vi "Get Service Descriptor.vi"(8 "error in":errorcluster) -> (0 "error out":errorcluster, 3 "service descriptor":T1)   [LabVIEW 2022 SP3, in "Single Tone - Digital Mic.lvlib"]
uses:
  Single Tone - Digital Mic.lvlib
  <vilib>/Plug-In SDKs/Measurements/Helpers/TypeDefs/Service Descriptor.ctl
  <vilib>/Plug-In SDKs/Measurements/Helpers/TypeDefs/Measurement Details.ctl
  <vilib>/Plug-In SDKs/Measurements/Helpers/TypeDefs/Measurement Annotation.ctl
  <vilib>/Plug-In SDKs/Measurements/NI Measurement Plug-In SDK.lvlib
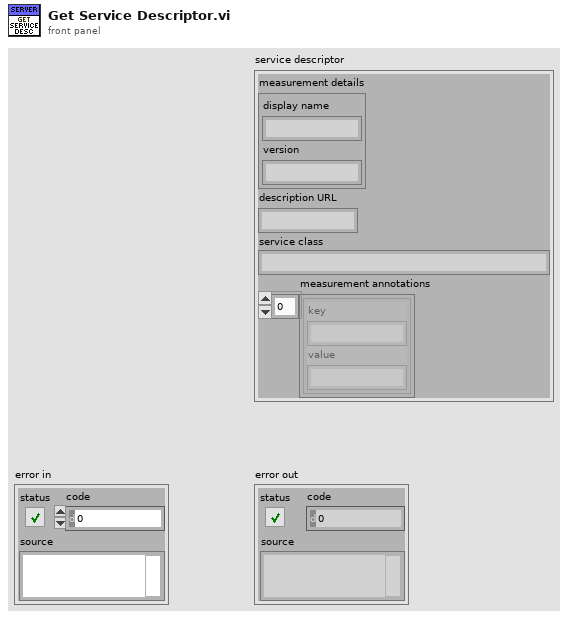
[diagram p1: front panel]
types:
  T1 = typedef "NI Measurement Plug-In SDK.lvlib/Service Descriptor.ctl" = cluster{"measurement details":T2, "description URL":string, "service class":string, "measurement annotations":T3[]}
  T2 = typedef "NI Measurement Plug-In SDK.lvlib/Measurement Details.ctl" = cluster{"display name":string, "version":string}
  T3 = typedef "NI Measurement Plug-In SDK.lvlib/Measurement Annotation.ctl" = cluster{"key":string, "value":string}
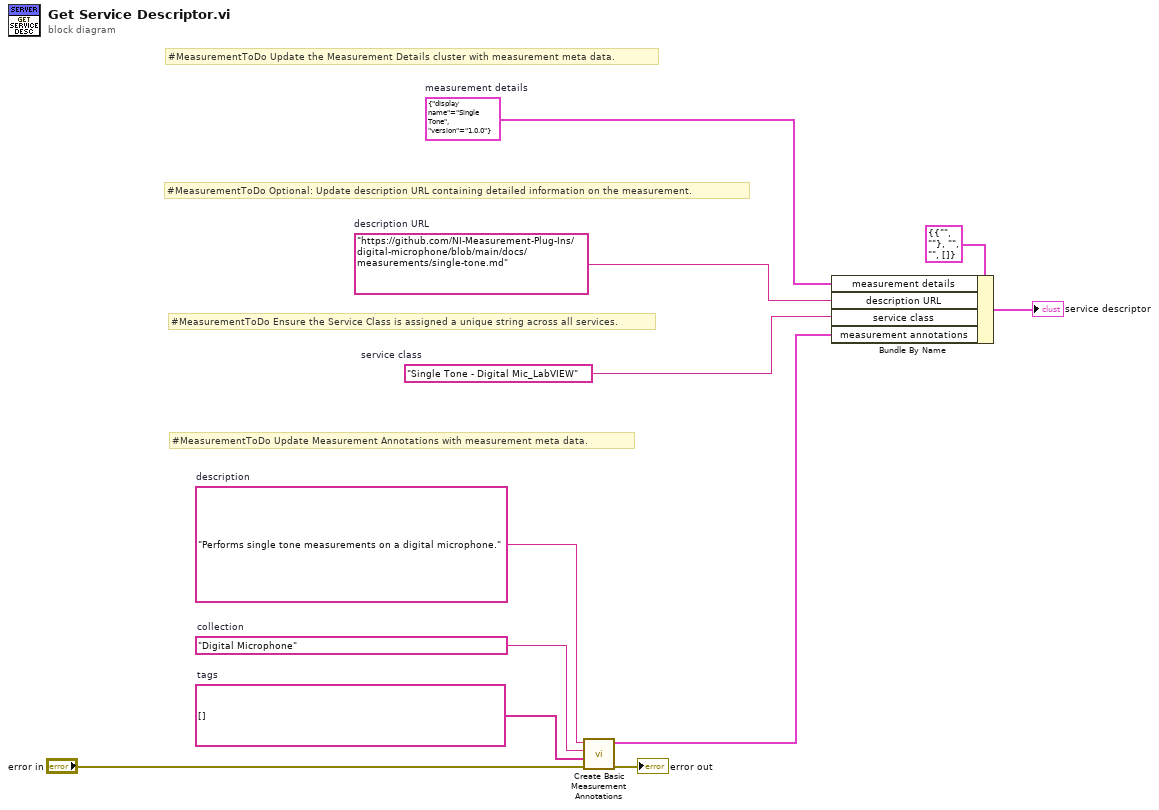
[diagram p0: block diagram]
diagram:
  w5 = "https://github.com/NI-Measurement-Plug-Ins/digital-microphone/blob/main/docs/measurements/single-tone.md"  # description URL
  w7 = string[] []  # tags
  w8 = "Digital Microphone"  # collection
  w9 = "Performs single tone measurements on a digital microphone."  # description
  w6 = T2 {"display name"="Single Tone", "version"="1.0.0"}  # measurement details
  w4 = "Single Tone - Digital Mic_LabVIEW"  # service class
  # "#MeasurementToDo Optional: Update description URL containing detailed information on the measurement."
  # "#MeasurementToDo Update Measurement Annotations with measurement meta data."
  # "#MeasurementToDo Ensure the Service Class is assigned a unique string across all services."
  # "#MeasurementToDo Update the Measurement Details cluster with measurement meta data."
  n1 = call <vilib>:"Create Basic Measurement Annotations.vi"("error in"="error in", "tags"=w7, "collection"=w8, "description"=w9) -> ("error out"=→"error out":errorcluster, "measurement annotations"=w3:T3[])  [unwired: 6 in]
  n2 = Bundle By Name(cluster=T1 {"measurement details"={"display name"="", "version"=""}, "description URL"="", "service class"="", "measurement annotations"=[]} ("service descriptor"), "measurement details"=w6, "description URL"=w5, "service class"=w4, "measurement annotations"=w3) -> (→"service descriptor":T1)
